vi "instantiate_data_pipeline.vi"(0 "sources":refnum<class "abstract_datasource_base.lvclass">[](array[class]), 5 "processing steps":refnum<class "abstract_dataprocessing_base.lvclass">[](array[class]), 7 "destinations":refnum<class "abstract_datadestination_base.lvclass">[](array[class]), 11 "error in (no error)":errorcluster) -> (4 "data_simple_pipeline out":refnum<class "data_simple_pipeline.lvclass">, 15 "error out":errorcluster)   [LabVIEW 2020, in "data_simple_pipeline.lvclass"]
uses:
  data_simple_pipeline.lvclass
  data_source/abstract_datasource_base/abstract_datasource_base.lvclass
  data_processor/abstract_dataprocessing_base/abstract_dataprocessing_base.lvclass
  data_destination/abstract_datadestination_base/abstract_datadestination_base.lvclass
  data_simple_pipeline.lvclass/data_simple_pipeline.ctl
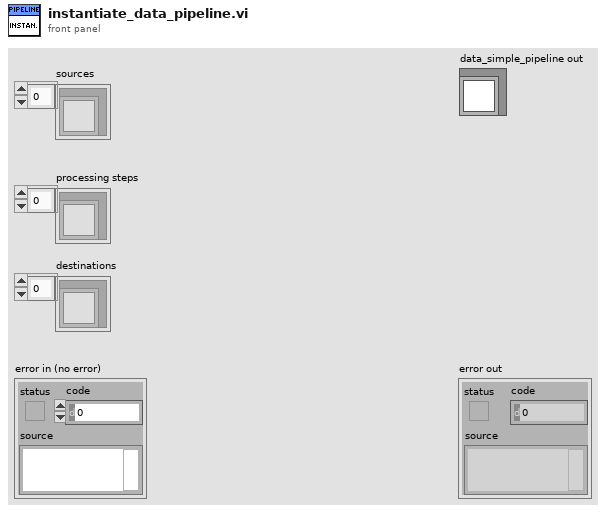
[diagram p1: front panel]
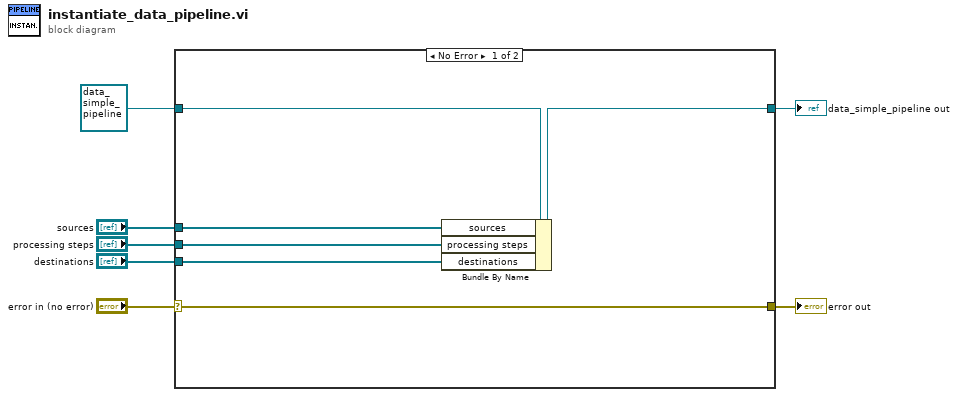
[diagram p0: block diagram]
diagram:
  n1 = case shown="No Error" "error in (no error)" {
    selector: "error in (no error)" -> [w13 w15]
    tunnel: [w13 w15] -> w6
    tunnel: [w8 w14] -> w4
    tunnel: refnum<class "data_simple_pipeline.lvclass"> refnum ("data_simple_pipeline in") -> [w12 w14]
    tunnel: "sources" -> [w11 _]
    tunnel: "processing steps" -> [w10 _]
    tunnel: "destinations" -> [w9 _]
    frame No Error {
      n2 = Bundle By Name(cluster=w12, "sources"=w11, "processing steps"=w10, "destinations"=w9) -> (w8:refnum<class "data_simple_pipeline.lvclass">)
    }
    frame Error {
    }
  }
  "error out" <- w6
  "data_simple_pipeline out" <- w4
